vi "Read Handle.vi"(8 "Error In":errorcluster, 11 "Listener In":refnum<class "Listener.lvclass">) -> (0 "Error Out":errorcluster, 2 "Handle":u64, 3 "Listener Out":refnum<class "Listener.lvclass">)   [LabVIEW 2018, in "Toolkit.lvlib" / "Listener.lvclass"]
uses:
  Listener.lvclass
  Listener.lvclass/Listener.ctl
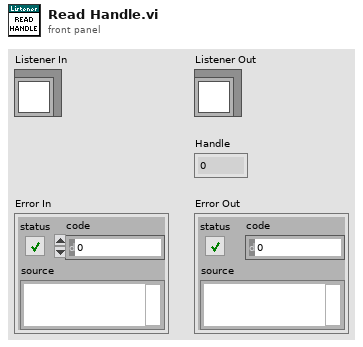
[diagram p1: front panel]
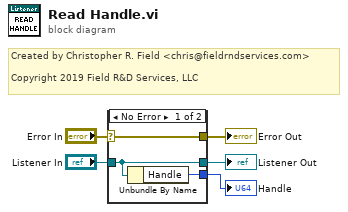
[diagram p0: block diagram]
diagram:
  # "Created by Christopher R. Field <chris@fieldrndservices.com>\n\nCopyright 2019 Field R&D Services, LLC"
  n1 = case shown="No Error" "Error In" {
    selector: "Error In" -> [w7 w10]
    tunnel: "Listener In" -> [w8 w9]
    tunnel: [w8 w9] -> w1
    tunnel: [w7 w10] -> w4
    tunnel: [w6 _] -> w3
    frame No Error {
      n2 = Unbundle By Name(w8) -> ("Handle"=w6:u64)
    }
    frame Error {
    }
  }
  "Error Out" <- w4
  "Handle" <- w3
  "Listener Out" <- w1
